vi "Select Class.vi"(8 "error in":errorcluster, 11 "Class Path":path=path "C:/GitHub/OOP Template/HAL/Concrete") -> (0 "error out":errorcluster, 3 "Class Ref":refnum<class>)   [LabVIEW 2019, in "Sequence Main.lvlib" / "Abstract UUT.lvclass"]
uses:
  Abstract UUT.lvclass
panel:
  in  "Abstract UUT":refnum<class "Abstract UUT.lvclass">
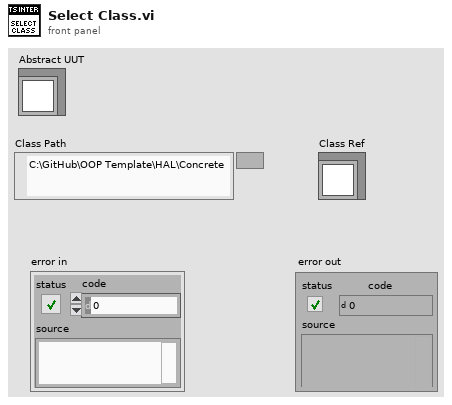
[diagram p1: front panel]
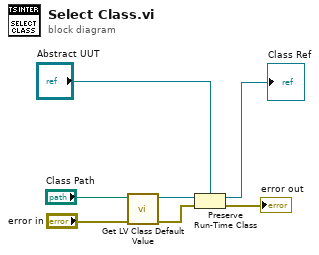
[diagram p0: block diagram]
diagram:
  n1 = call <vilib>:"Get LV Class Default Value.vi"("error in (no error)"="error in", "class path"="Class Path") -> ("error out"=w6:errorcluster, "object"=w2:refnum<class>)  [unwired: 8 in]
  n2 = Preserve Run-Time Class(object in=w2, error in=w6, 2:"Abstract UUT") -> (object out=→"Class Ref":refnum<class "Abstract UUT.lvclass">, error out=→"error out":errorcluster)
